vi "initialize.vi"(8 "error in (no error)":errorcluster, 11 "ModbusBuffer in":refnum<class "ModbusBuffer.lvclass">) -> (0 "error out":errorcluster, 3 "ModbusBuffer out":refnum<class "ModbusBuffer.lvclass">)   [LabVIEW 2016, in "RTModbus.lvlib" / "ModbusBuffer.lvclass"]
uses:
  ModbusBuffer.lvclass
  ModbusBuffer.lvclass/ModbusBuffer.ctl
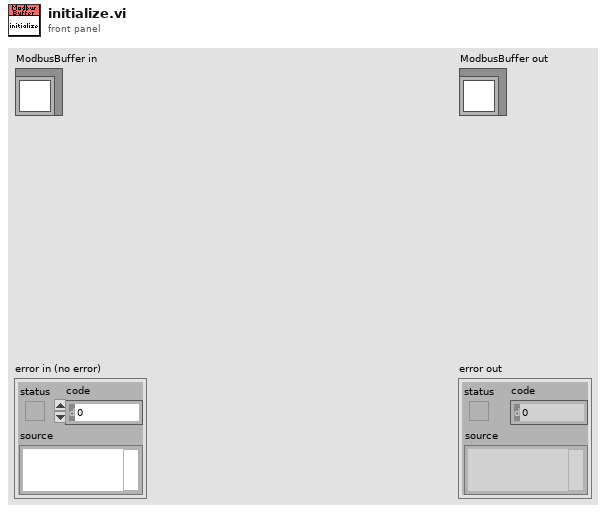
[diagram p1: front panel]
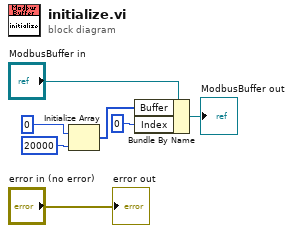
[diagram p0: block diagram]
diagram:
  n1 = Initialize Array(u16 0 ("element"), 20000 ("dimension size")) -> (w4:u16[])
  n2 = Bundle By Name(cluster="ModbusBuffer in", "Buffer"=w4, "Index"=0) -> (→"ModbusBuffer out":refnum<class "ModbusBuffer.lvclass">)
  "error out" <- "error in (no error)"
